vi "knife_edge_phase_,measurement.vi"() -> ()   [LabVIEW 2024]
panel:
  in  "SLM Queue":refnum<queue>
  in  "Modulation Mode":string
  in  "Y Shift B":i32
  in  "X Shift B":i32
  in  "A/B Display":bool
  in  "Use B Display":bool
  in  "Use A Display":bool
  in  "X/Y Shifting":bool
  in  "Y Shift A":i32
  in  "X Shift A":i32
  in  "Number of Shifts":i32
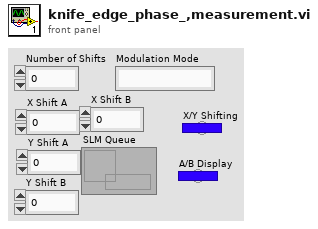
[diagram p1: front panel]
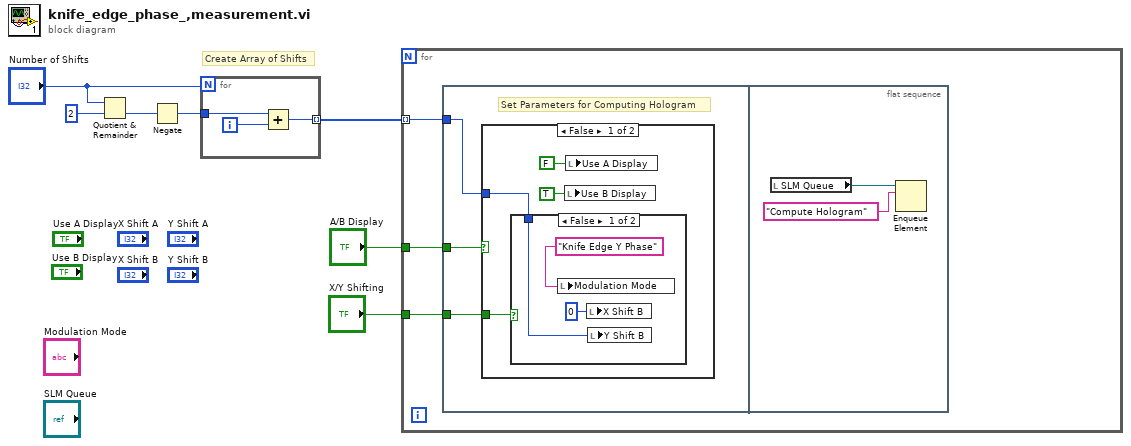
[diagram p0: block diagram]
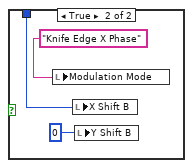
[diagram p2: hidden frame]
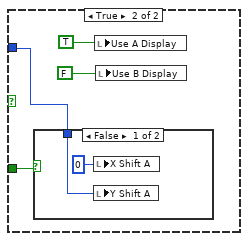
[diagram p3: hidden frame]
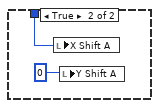
[diagram p4: hidden frame]
diagram:
  # "Create Array of Shifts"
  n1 = Quotient & Remainder(x="Number of Shifts", y=2) -> (floor(x/y)=w5:i32)  [unwired: 1 out]
  n2 = Negate(x=w5) -> (-x=w4:i32)
  n3 = for {
    N: "Number of Shifts" -> [_]
    tunnel: w4 -> [w10]
    tunnel: [w9] -> w3 mode=indexing
    i -> [w8]
    n4 = Add(x=w10, y=w8) -> (x+y=w9:i32)
  }
  n5 = for {
    tunnel: w3 -> [w13] mode=indexing
    tunnel: "A/B Display" -> [w12]
    tunnel: "X/Y Shifting" -> [w11]
    n6 = flat-sequence {
      tunnel: w13 -> [w16]
      tunnel: w12 -> [w15]
      tunnel: w11 -> [w14]
      frame #0 {
        # "Set Parameters for Computing Hologram"
        n7 = case shown="False" w15 {
          tunnel: w16 -> [w17 w27]
          tunnel: w14 -> [w18 w28]
          frame False {
            n8 = case shown="False" w18 {
              tunnel: w17 -> [w23 w26]
              frame False {
                n9 = local write "Modulation Mode"("Knife Edge Y Phase") -> ()
                n10 = local write "X Shift B"(0 ("X Shift B")) -> ()
                n11 = local write "Y Shift B"(w23) -> ()
              }
              frame True {
                n12 = local write "Modulation Mode"("Knife Edge X Phase") -> ()
                n13 = local write "X Shift B"(w26) -> ()
                n14 = local write "Y Shift B"(0) -> ()
              }
            }
            n15 = local write "Use B Display"(TRUE) -> ()
            n16 = local write "Use A Display"(FALSE) -> ()
          }
          frame True {
            n17 = case shown="False" w28 {
              tunnel: w27 -> [w32 w34]
              frame False {
                n18 = local write "X Shift A"(0) -> ()
                n19 = local write "Y Shift A"(w32) -> ()
              }
              frame True {
                n20 = local write "X Shift A"(w34) -> ()
                n21 = local write "Y Shift A"(0) -> ()
              }
            }
            n22 = local write "Use A Display"(TRUE) -> ()
            n23 = local write "Use B Display"(FALSE) -> ()
          }
        }
      }
      frame #1 {
        n24 = local read "SLM Queue"() -> (w36:refnum<queue>)
        n25 = Enqueue Element(queue=w36, element="Compute Hologram") -> ()  [unwired: 2 in, 3 out]
      }
    }
  }
